vi "Pow3.vi"(11 "x":i32) -> (3 "x^3":i32)   [LabVIEW 2013]
uses:
  Typedef/Powers of 3.ctl
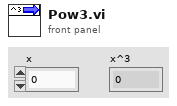
[diagram p1: front panel]
types:
  T1 = typedef "Powers of 3.ctl" = i32[]
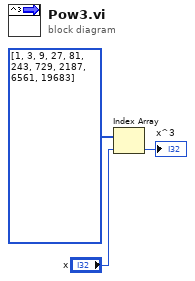
[diagram p0: block diagram]
diagram:
  n1 = Index Array(array=T1 [1, 3, 9, 27, 81, 243, 729, 2187, 6561, 19683], index="x") -> (element=→"x^3":i32)
